vi "Day 3.1 - Part Numbers.vi"(11 "input":string[](array[string])) -> (3 "ouptut part 1":u64)   [LabVIEW 2021]
uses:
  <vilib>/regexp/Match Regular Expression.xnode
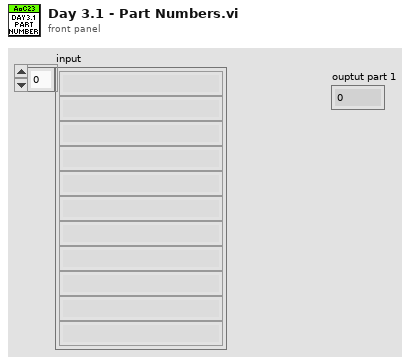
[diagram p1: front panel]
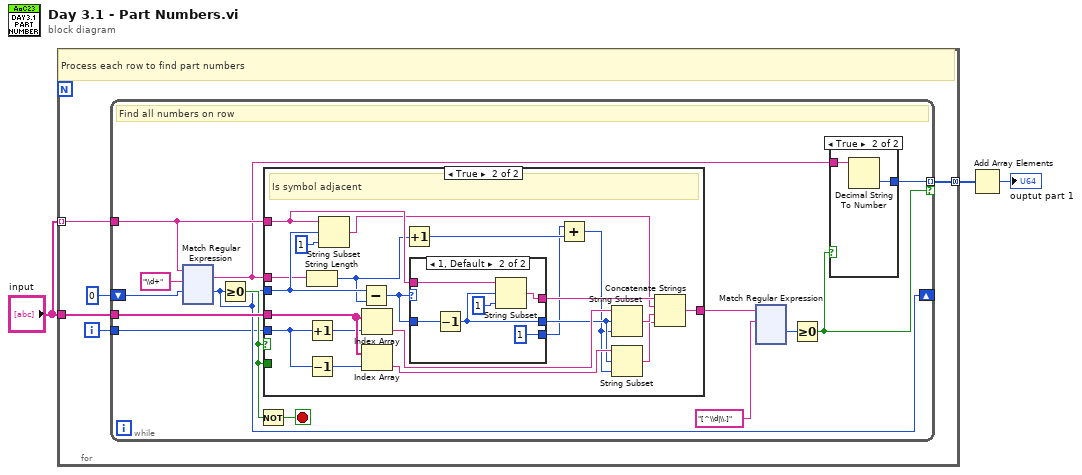
[diagram p0: block diagram]
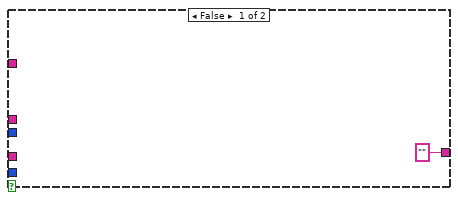
[diagram p3: hidden frame]
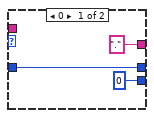
[diagram p4: hidden frame]
diagram:
  n1 = for {
    tunnel: "input" -> [w8] mode=indexing
    tunnel: "input" -> [w6]
    tunnel: [w4] -> w2 mode=concatenating
    i -> [w5]
    # "Process each row to find part numbers"
    n2 = while {
      tunnel: w8 -> [w18]
      tunnel: w6 -> [w19]
      shift-right: [w16] -> _
      shift-left: 0 -> [w20]
      tunnel: w5 -> [w15]
      tunnel: [w10] -> w4 mode=indexing if=w9
      stop <- w21 stop-if-true
      # "Find all numbers on row"
      n3 = xnode "Match Regular Expression"("input string"=w18, "regular expression"="\\d+", "offset (0)"=w20) -> ("whole match"=w11:string, "offset past match"=w16:i32)  [unwired: 3 in, 3 out]
      n4 = Greater Or Equal To 0?(x=w16) -> (x >= 0?=w17:bool)
      n5 = Not(x=w17) -> (.not. x?=w21:bool)
      n6 = case shown="True" w17 {
        tunnel: w11 -> [_ w156]
        tunnel: w17 -> [_ _]
        tunnel: w19 -> [_ w155]
        tunnel: w18 -> [_ w161]
        tunnel: ["" w163] -> w14
        tunnel: w16 -> [_ w158]
        tunnel: w15 -> [_ w152]
        frame False {
        }
        frame True {
          # "Is symbol adjacent"
          n7 = String Length(string=w156) -> (length=w145:i32)
          n8 = Increment(x=w152) -> (x+1=w154:i32)
          n9 = Decrement(x=w152) -> (x-1=w153:i32)
          n10 = String Subset(string=w161, offset (0)=w158, length (rest)=1 ("length (rest)")) -> (substring=w159:string)
          n11 = Subtract(x=w158, y=w145) -> (x-y=w157:i32)
          n12 = Index Array(array=w155, index=w154) -> (element=w151:string)
          n13 = Index Array(array=w155, index=w153) -> (element=w150:string)
          n14 = Increment(x=w145) -> (x+1=w149:i32)
          n15 = case shown="1, Default" w157 {
            tunnel: w161 -> [_ w172]
            tunnel: w157 -> [w165 w171]
            tunnel: ["." w169] -> w160
            tunnel: [w165 w168] -> w146
            tunnel: [0 1] -> w143
            frame 0 {
            }
            frame 1, Default {
              n16 = Decrement(x=w171) -> (x-1=w168:i32)
              n17 = String Subset(string=w172, offset (0)=w168, length (rest)=1 ("length (rest)")) -> (substring=w169:string)
            }
          }
          n18 = Add(x=w143, y=w149) -> (x+y=w144:i32)
          n19 = String Subset(string=w151, offset (0)=w146, length (rest)=w144) -> (substring=w148:string)
          n20 = String Subset(string=w150, offset (0)=w146, length (rest)=w144) -> (substring=w147:string)
          n21 = Concatenate Strings(w160, w159, w148, w147) -> (w163:string)
        }
      }
      n22 = xnode "Match Regular Expression"("input string"=w14, "regular expression"="[^\\d|\\.]") -> ("offset past match"=w12:i32)  [unwired: 4 in, 4 out]
      n23 = Greater Or Equal To 0?(x=w12) -> (x >= 0?=w9:bool)
      n24 = case shown="True" w9 {
        tunnel: w11 -> [_ w24]
        tunnel: [_ w23] -> w10
        frame False {
        }
        frame True {
          n25 = Decimal String To Number(string=w24) -> (number=w23:i32)  [unwired: 2 in, 1 out]
        }
      }
    }
  }
  n26 = Add Array Elements(numeric array=w2) -> (sum=→"ouptut part 1":i32)
